vi "Configure Period.vi"(8 "error in (no error)":errorcluster, 9 "Period Estimate (100E-9s)":dbl=1e-07 format="%^#_7g", 11 "VISA resource name":refnum<visa-resource-name>) -> (0 "error out":errorcluster, 3 "VISA resource name out":refnum<visa-resource-name>)   [LabVIEW 2020, in "Counter.lvlib" / "PICOTEST U62XXA series.lvlib"]
doc: "Configures the parameters required for Period measurements.\n\n<B>Note:</B>\nThe U6220A model <B>does not</B> provide the channel 2 & 3.\n\nThe measurement arming is coupled to Digits. Arming can be changed by calling any of the Arming VIs. The measurement channel has auto-trigger enabled at 50% with a positive slope."
uses:
  PICOTEST U62XXA series.lvlib
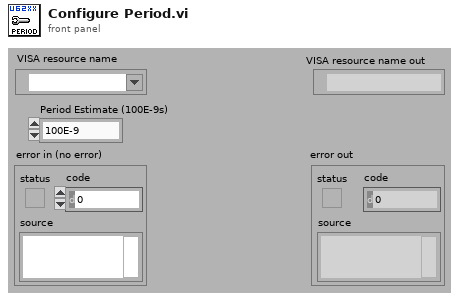
[diagram p1: front panel]
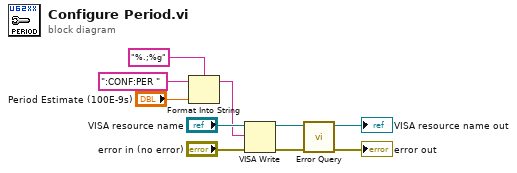
[diagram p0: block diagram]
diagram:
  n1 = Format Into String(format string="%.;%g", initial string=":CONF:PER ", "Period Estimate (100E-9s)") -> (resulting string=w5:string)  [unwired: 1 in, 1 out]
  n2 = VISA Write(VISA resource name="VISA resource name", write buffer=w5, error in (no error)="error in (no error)") -> (VISA resource name out=w4:refnum<visa-resource-name>, error out=w2:errorcluster)  [unwired: 1 out]
  n3 = call "Error Query.vi"("error in (no error)"=w2, "VISA resource name"=w4) -> ("error out"=→"error out":errorcluster, "VISA resource name out"=→"VISA resource name out":refnum<visa-resource-name>)  [unwired: 6 in, 2 out]
